vi "RANK.vi"(1 "3*3陣列":string[][](array[string])) -> (0 "O┪X墓":bool)   [LabVIEW 2014]
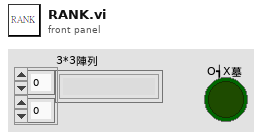
[diagram p1: front panel]
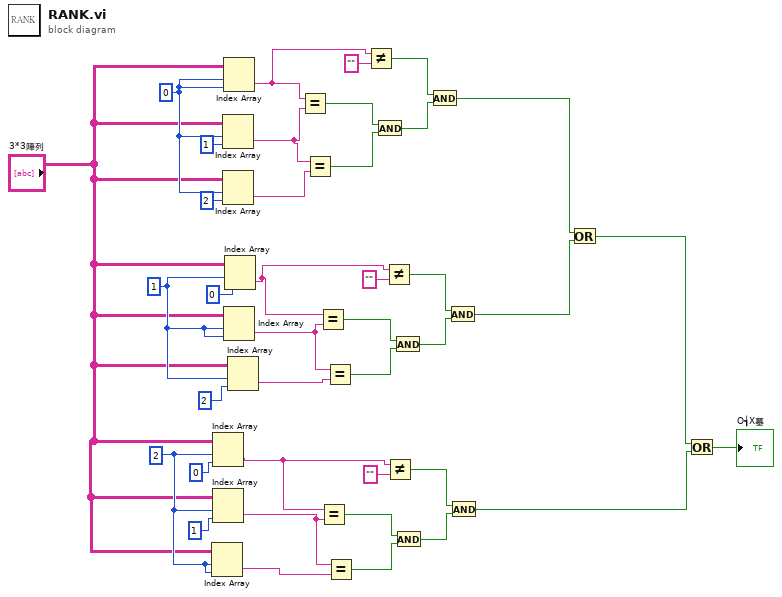
[diagram p0: block diagram]
diagram:
  w17 = 2
  w28 = 1
  w39 = 0
  n1 = Index Array(array="3*3陣列", index (row)=w17, index (col)=w17) -> (element=w6:string)
  n2 = Index Array(array="3*3陣列", index (row)=w17, index (col)=0) -> (element=w8:string)
  n3 = Index Array(array="3*3陣列", index (row)=w17, index (col)=1) -> (element=w7:string)
  n4 = Index Array(array="3*3陣列", index (row)=w39, index (col)=1) -> (element=w36:string)
  n5 = Index Array(array="3*3陣列", index (row)=w39, index (col)=2) -> (element=w35:string)
  n6 = Index Array(array="3*3陣列", index (row)=w39, index (col)=w39) -> (element=w31:string)
  n7 = Index Array(array="3*3陣列", index (row)=w28, index (col)=w28) -> (element=w19:string)
  n8 = Index Array(array="3*3陣列", index (row)=w28, index (col)=0) -> (element=w20:string)
  n9 = Index Array(array="3*3陣列", index (row)=w28, index (col)=2) -> (element=w18:string)
  n10 = Equal?(x=w31, y=w36) -> (x = y?=w34:bool)
  n11 = Equal?(x=w36, y=w35) -> (x = y?=w33:bool)
  n12 = Equal?(x=w20, y=w19) -> (x = y?=w25:bool)
  n13 = Equal?(x=w8, y=w7) -> (x = y?=w13:bool)
  n14 = Equal?(x=w19, y=w18) -> (x = y?=w24:bool)
  n15 = Equal?(x=w7, y=w6) -> (x = y?=w12:bool)
  n16 = Not Equal?(x=w31, y="") -> (x != y?=w30:bool)
  n17 = And(x=w34, y=w33) -> (x .and. y?=w29:bool)
  n18 = Not Equal?(x=w20, y="") -> (x != y?=w22:bool)
  n19 = Not Equal?(x=w8, y="") -> (x != y?=w10:bool)
  n20 = And(x=w25, y=w24) -> (x .and. y?=w21:bool)
  n21 = And(x=w13, y=w12) -> (x .and. y?=w9:bool)
  n22 = And(x=w30, y=w29) -> (x .and. y?=w5:bool)
  n23 = And(x=w22, y=w21) -> (x .and. y?=w4:bool)
  n24 = And(x=w10, y=w9) -> (x .and. y?=w3:bool)
  n25 = Or(x=w5, y=w4) -> (x .or. y?=w2:bool)
  n26 = Or(x=w2, y=w3) -> (x .or. y?=→"O┪X墓":bool)
